vi "Calculate Differences.vi"(10 "Actual":dbl[](array[numeric]), 11 "Setpoint":dbl[](array[numeric])) -> (3 "Pod Comparisons (Diff -> Setpoint - Actual)":T1)   [LabVIEW 2020]
uses:
  <vilib>/Analysis/coordinate.llb/Angle Range (Degree).ctl
  <vilib>/Analysis/coordinate.llb/Angle Units.ctl
  <vilib>/Analysis/coordinate.llb/Wrap Angle (scalar).vi
  <vilib>/Analysis/NI_AAL_Angle.lvlib
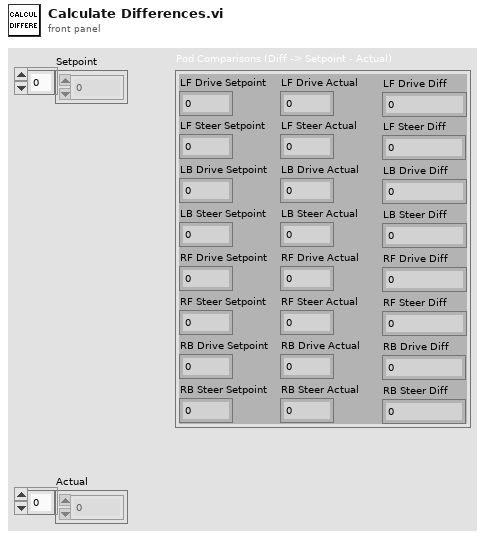
[diagram p1: front panel]
types:
  T1 = cluster{"LF Drive Setpoint":dbl, "LF Steer Setpoint":dbl, "LB Drive Setpoint":dbl, "LB Steer Setpoint":dbl, "RF Drive Setpoint":dbl, "RF Steer Setpoint":dbl, "RB Drive Setpoint":dbl, "RB Steer Setpoint":dbl, "LF Drive Actual":dbl, "LF Steer Actual":dbl, "LB Drive Actual":dbl, "LB Steer Actual":dbl, "RF Drive Actual":dbl, "RF Steer Actual":dbl, "RB Drive Actual":dbl, "RB Steer Actual":dbl, "LF Drive Diff":dbl, "LF Steer Diff":dbl, "LB Drive Diff":dbl, "LB Steer Diff":dbl, "RF Drive Diff":dbl, "RF Steer Diff":dbl, "RB Drive Diff":dbl, "RB Steer Diff":dbl}
  T2 = typedef "NI_AAL_Angle.lvlib/Angle Units.ctl" = i32
  T3 = typedef "NI_AAL_Angle.lvlib/Angle Range (Degree).ctl" = u16
  T4 = cluster{"[0]":dbl, "[1]":dbl, "[2]":dbl, "[3]":dbl, "[4]":dbl, "[5]":dbl, "[6]":dbl, "[7]":dbl, "[8]":dbl, "[9]":dbl, "[10]":dbl, "[11]":dbl, "[12]":dbl, "[13]":dbl, "[14]":dbl, "[15]":dbl, "[16]":dbl, "[17]":dbl, "[18]":dbl, "[19]":dbl, "[20]":dbl, "[21]":dbl, "[22]":dbl, "[23]":dbl}
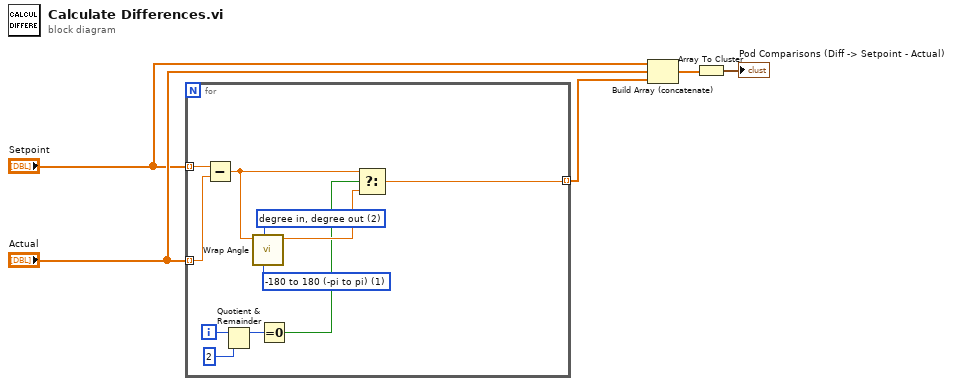
[diagram p0: block diagram]
diagram:
  n1 = for {
    tunnel: "Setpoint" -> [w13] mode=indexing
    tunnel: "Actual" -> [w12] mode=indexing
    tunnel: [w6] -> w3 mode=indexing
    i -> [w16]
    w9 = T2 2 items=["radian in, radian out", "radian in, degree out", "degree in, degree out", "degree in, radian out"] ("angle units")
    w10 = T3 1 items=["none", "-180 to 180 (-pi to pi)", "0 to 360 (0 to 2pi)"] ("angle range")
    n2 = Subtract(x=w13, y=w12) -> (x-y=w11:dbl)
    n3 = Quotient & Remainder(x=w16, y=2) -> (x-y*floor(x/y)=w14:i32)  [unwired: 1 out]
    n4 = call-poly <vilib>:"Wrap Angle.vi"("angle units"=w9, "angle range"=w10, "angle in"=w11) -> ("angle out"=w8:dbl)  [unwired: 7 in, 1 out]
    n5 = Equal To 0?(x=w14) -> (x = 0?=w7:bool)
    n6 = Select(t=w11, s=w7, f=w8) -> (s? t:f=w6:dbl)
  }
  n7 = Build Array (concatenate)("Setpoint", "Actual", w3) -> (w1:dbl[])
  n8 = Array To Cluster(array=w1) -> (cluster=→"Pod Comparisons (Diff -> Setpoint - Actual)":T4)
